vi "Server_Registering.vi"(8 "error in":errorcluster, 11 "User Data":T2={"Name"="Guset", "Email"="", "Phone Number"="", "User Picture"=array225x225[50625 elements], "Last Login Time"=timestamp(0 s since 1904-01-01)}) -> (0 "error out":errorcluster, 3 "User Registering Status":T1)   [LabVIEW 2018, in "Cloud Server.lvlib"]
uses:
  Cloud Server.lvlib
  Com VIs/Data Def/User Data.ctl
  Com VIs/Data Def/User Registering Status.ctl
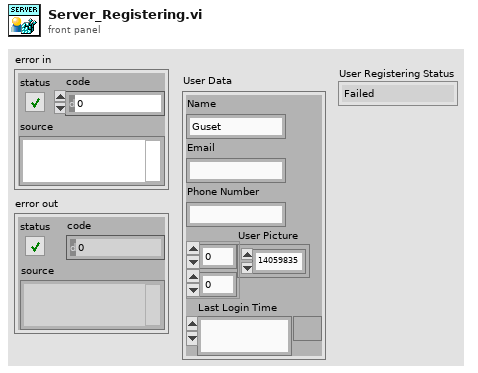
[diagram p1: front panel]
types:
  T1 = typedef "User Registering Status.ctl" = enum16{"Failed", "Duplicate", "Success"}
  T2 = typedef "User Data.ctl" = cluster{"Name":string, "Email":string, "Phone Number":string, "User Picture":u32[][], "Last Login Time":timestamp}
  T3 = enum16{"open", "replace", "create", "open or create", "replace or create", "replace or create with confirmation"}
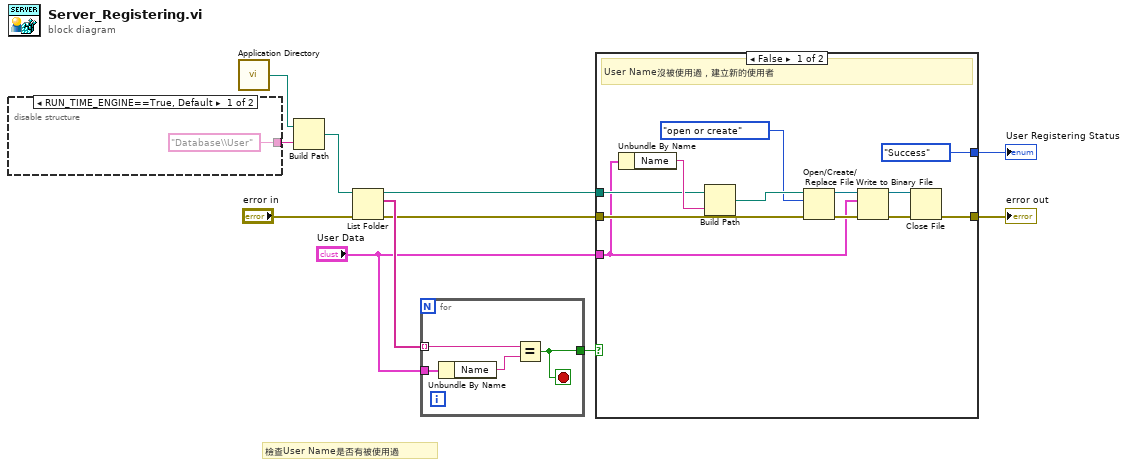
[diagram p0: block diagram]
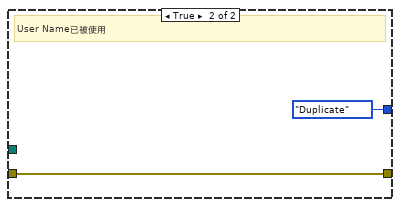
[diagram p2: hidden frame]
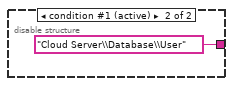
[diagram p3: hidden frame]
diagram:
  # "檢查User Name是否有被使用過"
  n1 = disable-structure shown="RUN_TIME_ENGINE==True, Default" {
    disable-tunnel: ["Database\\User" ("name or relative path") "Cloud Server\\Database\\User" ("name or relative path")] -> w11
    frame condition #0 {
    }
    frame condition #1 (active) {
    }
  }
  n2 = call <vilib>:"Application Directory.vi"() -> ("Application Directory"=w10:path)
  n3 = Build Path(base path=w10, name or relative path=w11) -> (appended path=w9:path)
  n4 = List Folder(path=w9, error in="error in") -> (path out=w4:path, filenames=w7:string[], error out=w6:errorcluster)  [unwired: 2 in, 1 out]
  n5 = for {
    tunnel: [w17] -> w5
    tunnel: w7 -> [w16] mode=indexing
    tunnel: "User Data" -> [w15]
    stop <- w17 stop-if-true
    n6 = Unbundle By Name(w15) -> ("Name"=w14:string)
    n7 = Equal?(x=w16, y=w14) -> (x = y?=w17:bool)
  }
  n8 = case shown="False" w5 {
    tunnel: w6 -> [w29 w31]
    tunnel: w4 -> [w27 _]
    tunnel: "User Data" -> [w22 _]
    tunnel: [w19 w31] -> w1
    tunnel: [User_Registering_Status."Success" ("User Registering Status") User_Registering_Status."Duplicate" ("User Registering Status")] -> w2
    frame False {
      # "User Name沒被使用過，建立新的使用者"
      n9 = Unbundle By Name(w22) -> ("Name"=w28:string)
      n10 = Build Path(base path=w27, name or relative path=w28) -> (appended path=w26:path)
      n11 = Open/Create/Replace File(file path (use dialog)=w26, error in=w29, operation (0:open)=T3."open or create") -> (refnum out=w23:refnum<file>, error out=w24:errorcluster)  [unwired: 3 in, 1 out]
      n12 = Write to Binary File(file (use dialog)=w23, data=w22, error in=w24) -> (refnum out=w20:refnum<file>, error out=w21:errorcluster)  [unwired: 3 in, 1 out]
      n13 = Close File(refnum=w20, error in=w21) -> (error out=w19:errorcluster)  [unwired: 1 out]
    }
    frame True {
      # "User Name已被使用"
    }
  }
  "error out" <- w1
  "User Registering Status" <- w2
